vi "epen-ecu.vi"() -> ()   [LabVIEW 2015]
uses:
  M208910/class.dbc/controls/ecu-s.ctl
  <vilib>/xnet/xnet.llb/XNET String To IO Name (Database Alias).vi
  <resource>/objmgr/xnet.rc
panel:
  out "Array":T1[](array[typedef])
  out "Cluster 2":T1
  out "ECUs":refnum<k21>[][](array[refnum])
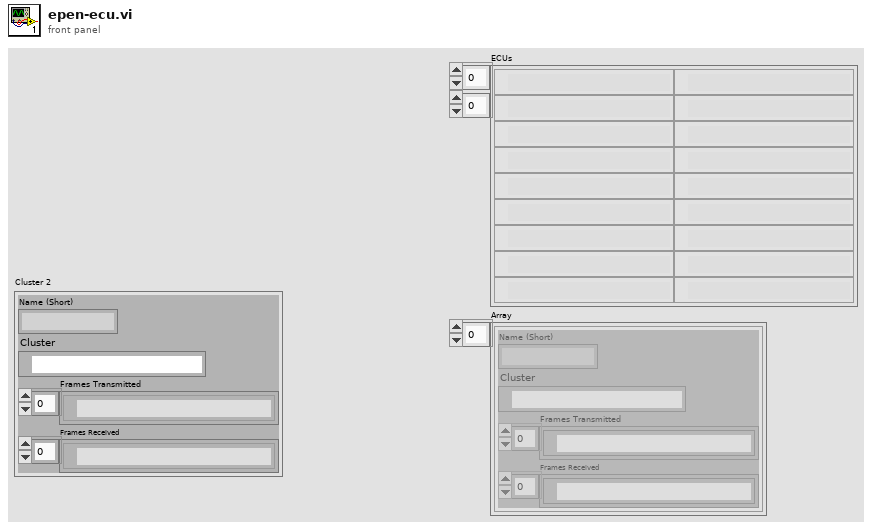
[diagram p1: front panel]
types:
  T1 = typedef "ecu-s.ctl" = cluster{"Name (Short)":string, "Cluster":refnum<k21>, "Frames Transmitted":refnum<k21>[], "Frames Received":refnum<k21>[]}
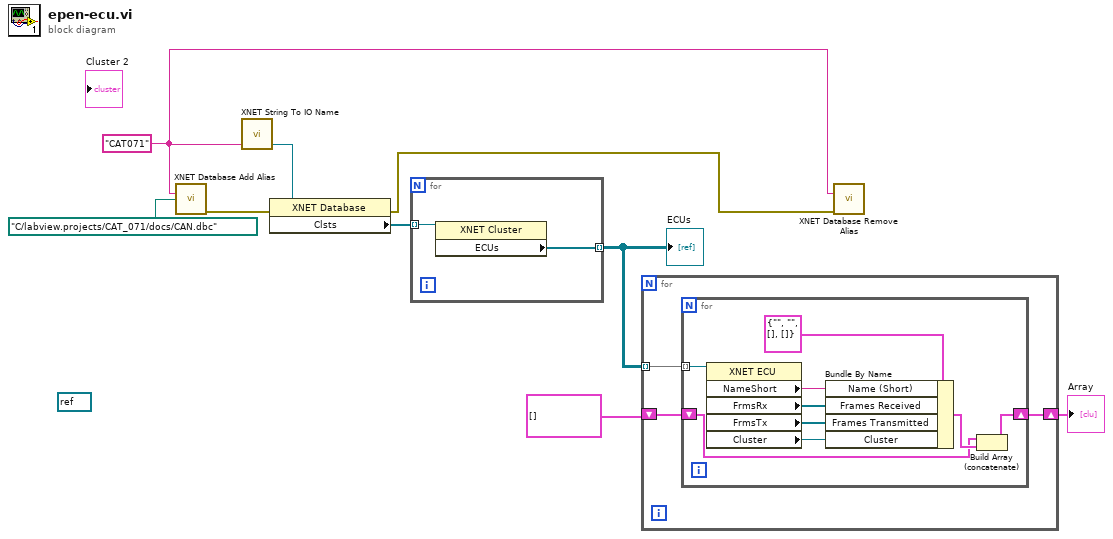
[diagram p0: block diagram]
diagram:
  (unwired) refnum<k21> refnum ("XNET Database")
  w8 = "CAT071" ("string")
  n1 = call <vilib>:"XNET Database Add Alias.vi"("alias"=w8, "filepath"=path "C:/labview.projects/CAT_071/docs/CAN.dbc" ("Path")) -> ("error out"=w7:errorcluster)  [unwired: 13 in]
  n2 = call-poly <vilib>:"XNET String To IO Name.vi"("string"=w8) -> ("XNET Database"=w6:refnum<k21>)  [unwired: 4 out]
  n3 = property class="XNET Database"(reference=w6, error in=w7) -> (error out=w4:errorcluster, "Clsts"=w5:refnum<k21>[])  [unwired: 1 out]
  n4 = for {
    tunnel: w5 -> [w11] mode=indexing
    tunnel: [w10] -> w3 mode=indexing
    n5 = property class="XNET Cluster"(reference=w11) -> ("ECUs"=w10:refnum<k21>[])  [unwired: 1 in, 2 out]
  }
  "ECUs" <- w3
  n6 = for {
    tunnel: w3 -> [w14] mode=indexing
    shift-right: [w12] -> w1
    shift-left: T1[] [] -> [w13]
    n7 = for {
      tunnel: w14 -> [w23] mode=indexing
      shift-right: [w16] -> w12
      shift-left: w13 -> [w15]
      n8 = property class="XNET ECU"(reference=w23) -> ("NameShort"=w21:string, "FrmsRx"=w20:refnum<k21>[], "FrmsTx"=w19:refnum<k21>[], "Cluster"=w18:refnum<k21>)  [unwired: 1 in, 2 out]
      n9 = Bundle By Name(cluster=T1 {"Name (Short)"="", "Cluster"="", "Frames Transmitted"=[], "Frames Received"=[]} ("ecus"), "Name (Short)"=w21, "Frames Received"=w20, "Frames Transmitted"=w19, "Cluster"=w18) -> (w17:T1)
      n10 = Build Array (concatenate)(w15, w17) -> (w16:T1[])
    }
  }
  "Array" <- w1
  n11 = call <vilib>:"XNET Database Remove Alias.vi"("alias"=w8, "error in (no error)"=w4) -> ()  [unwired: 13 in, 1 out]
